vi "Init.vi"(9 "Payload":T6, 10 "MsgExecuteType":T1, 11 "Priority":bool) -> (3 "Msg":T2 {"MsgAttribs"."AbsoluteTime" format="%<%x %.3X>T"})   [LabVIEW 2020, in "_Template.lvlib" / "{{Msg}}.lvlib"]
uses:
  {{Msg}}.lvlib
  Msg/Msg.lvclass
  jettl/jettl/Origin.ctl
  jettl/jettl/jettl.lvlib
  jettl/jettl/MsgAttribs.ctl
  jettl/jettl/Metadata/Metadata.lvclass
  jettl/jettl/Lifecycle.ctl
  jettl/jettl/Msg/Msg.lvclass
  jettl/jettl/Msg.ctl
  jettl/jettl/MsgExecuteType.ctl
  Payload.ctl
panel:
  # "This front panel should not be manipulated."
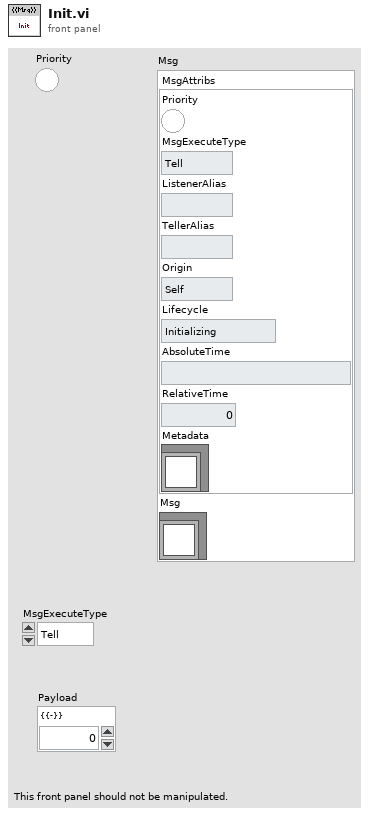
[diagram p1: front panel]
types:
  T1 = typedef "jettl.lvlib/MsgExecuteType.ctl" = enum16{"Tell", "Call"}
  T2 = typedef "jettl.lvlib/Msg.ctl" = cluster{"MsgAttribs":T3, "Msg":refnum<class "Msg.lvclass">}
  T3 = typedef "jettl.lvlib/MsgAttribs.ctl" = cluster{"Priority":bool, "MsgExecuteType":T1, "ListenerAlias":string, "TellerAlias":string, "Origin":T4, "Lifecycle":T5, "AbsoluteTime":timestamp, "RelativeTime":dbl, "Metadata":refnum<class "Metadata.lvclass">}
  T4 = typedef "jettl.lvlib/Origin.ctl" = enum16{"Self", "Parent", "Child"}
  T5 = typedef "jettl.lvlib/Lifecycle.ctl" = enum16{"Initializing", "SettingUp", "Starting", "Running", "Stopping", "TearingDown", "Terminated"}
  T6 = typedef "_Template.lvlib/{{Msg}}.lvlib/Payload.ctl" = cluster{"{{-}}":u8}
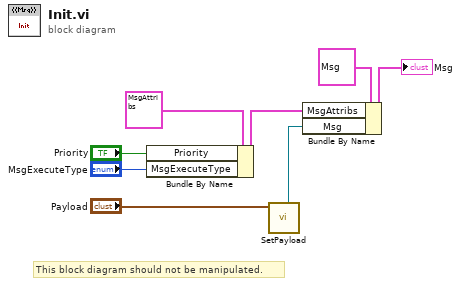
[diagram p0: block diagram]
diagram:
  # "This block diagram should not be manipulated."
  n1 = Bundle By Name(cluster=T3 {"Priority"=FALSE, "MsgExecuteType"=enum."Tell", "ListenerAlias"="", "TellerAlias"="", "Origin"=enum."Self", "Lifecycle"=enum."Initializing", "AbsoluteTime"=timestamp(0 s since 1904-01-01), "RelativeTime"=0.0, "Metadata"=refnum} ("Metadata"), "Priority"="Priority", "MsgExecuteType"="MsgExecuteType") -> (w1:T3)
  n2 = call "SetPayload.vi"("Payload"="Payload") -> ("Msg"=w6:refnum<class "Msg.lvclass">)  [unwired: 10 in]
  n3 = Bundle By Name(cluster=T2 {"MsgAttribs"={"Priority"=FALSE, "MsgExecuteType"=enum."Tell", "ListenerAlias"="", "TellerAlias"="", "Origin"=enum."Self", "Lifecycle"=enum."Initializing", "AbsoluteTime"=timestamp(0 s since 1904-01-01), "RelativeTime"=0.0, "Metadata"=refnum}, "Msg"=refnum} ("Msg"), "MsgAttribs"=w1, "Msg"=w6) -> (→"Msg":T2)
